vi "Points to Oval.vi"(0 "Image In":T2, 1 "Point":T1 {"Y Centroids" format="%.2f"; "X Centroids" format="%.2f"}, 2 "Size":dbl) -> (3 "Image Out":T2(plugin-control))   [LabVIEW 2015]
uses:
  <vilib>/vision/Image Controls.llb/IMAQ Image.ctl
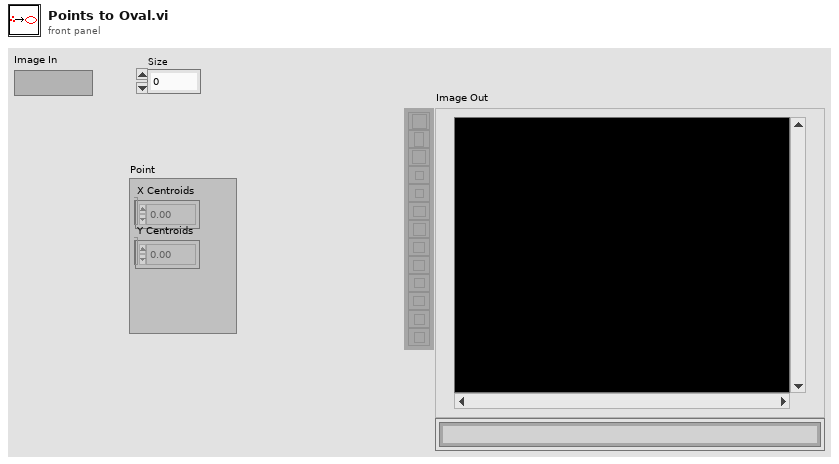
[diagram p1: front panel]
types:
  T1 = cluster{"X Centroids":sgl[], "Y Centroids":sgl[]}
  T2 = typedef "IMAQ Image.ctl" = refnum<image>
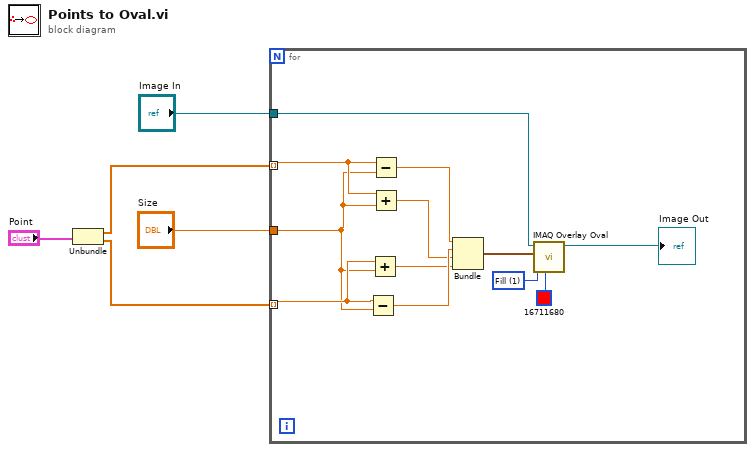
[diagram p0: block diagram]
diagram:
  n1 = Unbundle("Point") -> ("X Centroids"=w2:sgl[], "Y Centroids"=w1:sgl[])
  n2 = for {
    tunnel: w2 -> [w15] mode=indexing
    tunnel: w1 -> [w13] mode=indexing
    tunnel: "Size" -> [w11]
    tunnel: "Image In" -> [w8]
    w6 = u32 1 items=["Frame", "Fill"] ("Drawing Mode (Frame)")
    n3 = Subtract(x=w13, y=w11) -> (x-y=w16:dbl)
    n4 = Add(x=w13, y=w11) -> (x+y=w12:dbl)
    n5 = Subtract(x=w15, y=w11) -> (x-y=w17:dbl)
    n6 = Add(x=w15, y=w11) -> (x+y=w14:dbl)
    n7 = Bundle(w17, w16, w14, w12) -> (w10:cluster{dbl, dbl, dbl, dbl})  [unwired: 1 in]
    n8 = call "IMAQ Overlay Oval"("Color"=u32 16711680, "Drawing Mode (Frame)"=w6, "Bounding Rectangle"=w10, "Image"=w8) -> ("Image Out"=→"Image Out":T2)  [unwired: 6 in, 1 out]
  }
